vi "Conditionally Add Parity Parameter.vi"(10 "create parity (F)":bool, 11 "parameters in":T1[](array[typedef])) -> (3 "parameters out":T1[](array[typedef]))   [LabVIEW 2020]
uses:
  VS Channel Definition for Parameter.ctl
  Parameter Definition.ctl
  <vilib>/NI/NI VeriStand Encoding and Decoding/Encoding.ctl
  <vilib>/NI/NI VeriStand Encoding and Decoding/Encoding and Decoding.lvlib
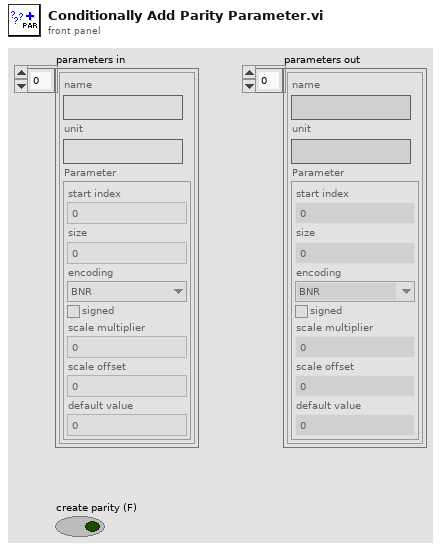
[diagram p1: front panel]
types:
  T1 = typedef "VS Channel Definition for Parameter.ctl" = cluster{"name":string, "unit":string, "Parameter":T2}
  T2 = typedef "Parameter Definition.ctl" = cluster{"start index":i32, "size":i32, "encoding":T3, "signed":bool, "scale multiplier":dbl, "scale offset":dbl, "default value":dbl}
  T3 = typedef "Encoding and Decoding.lvlib/Encoding.ctl" = enum16{"BNR", "BCD", "Discrete"}
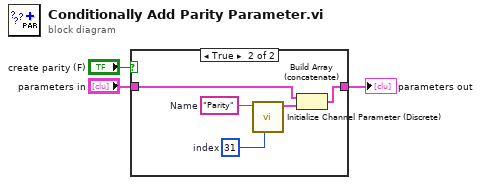
[diagram p0: block diagram]
diagram:
  n1 = case shown="True" "create parity (F)" {
    tunnel: "parameters in" -> [w4 w9]
    tunnel: [w4 w8] -> w2
    frame False {
    }
    frame True {
      w5 = 31  # index
      w6 = "Parity"  # Name
      n2 = call "Initialize Channel Parameter (Discrete).vi"("index"=w5, "name"=w6) -> ("channel parameter"=w7:T1)  [unwired: 9 in]
      n3 = Build Array (concatenate)(w9, w7) -> (w8:T1[])
    }
  }
  "parameters out" <- w2
